vi "Write Multi Channel U8 1D Array.vi"(8 "error in (no error)":errorcluster, 10 "Multi Channel U8 1D Array":u8[](array[numeric]), 11 "Model Driver in":refnum<class "Model Driver.lvclass">) -> (0 "error out":errorcluster, 3 "Model Driver out":refnum<class "Model Driver.lvclass">)   [LabVIEW 2023, in "Model Driver.lvclass"]
uses:
  Model Driver.lvclass
  Model Driver.lvclass/Model Driver.ctl
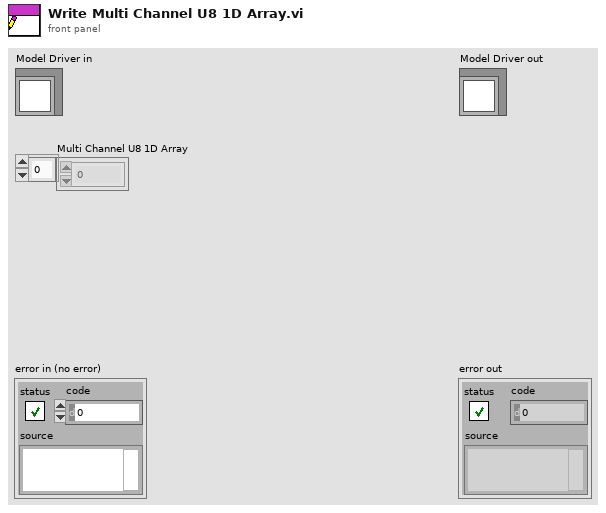
[diagram p1: front panel]
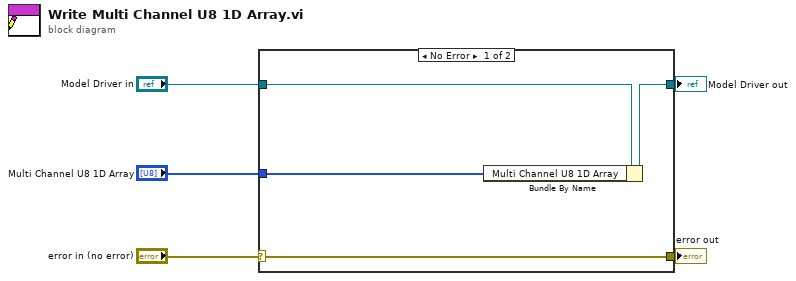
[diagram p0: block diagram]
diagram:
  n1 = case shown="No Error" "error in (no error)" {
    selector: "error in (no error)" -> [w9 w10]
    tunnel: [w9 w10] -> w4
    tunnel: [w7 w11] -> w2
    tunnel: "Model Driver in" -> [w8 w11]
    tunnel: "Multi Channel U8 1D Array" -> [w6 _]
    frame No Error {
      n2 = Bundle By Name(cluster=w8, "Multi Channel U8 1D Array"=w6) -> (w7:refnum<class "Model Driver.lvclass">)
    }
    frame Error {
    }
  }
  "error out" <- w4
  "Model Driver out" <- w2
